vi "create.mcap_id.vi"(10 "id":i32) -> (3 "Timestamp Manifest":refnum<class "mcap.lvclass">)   [LabVIEW 2020, in "nominal types.lvlib" / "timestampManifest.lvlib"]
uses:
  timestampManifest.lvlib
  mcap/mcap.lvclass
  id/id.lvclass
  C:/code/labview-client/lv_src/nominal types/filterTypes/filterTypes.lvclass
  C:/code/labview-client/lv_src/Nominal Client/datasources/payload/payload.lvclass
  C:/code/labview-client/lv_src/nominal types/id/id.lvclass
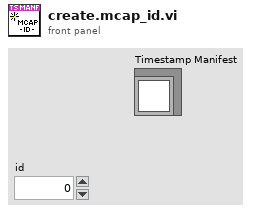
[diagram p1: front panel]
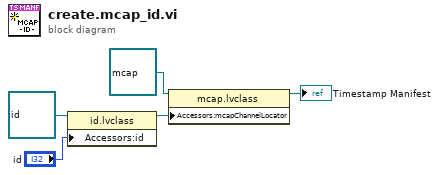
[diagram p0: block diagram]
diagram:
  n1 = property class="id.lvclass"(reference=refnum<class "id.lvclass"> refnum ("nominal types.lvlib:channelFilter.lvlib:id.lvclass"), "Accessors:id"="id") -> (reference out=w2:refnum<class "id.lvclass">)  [unwired: 1 in, 1 out]
  n2 = property class="mcap.lvclass"(reference=refnum<class "mcap.lvclass"> refnum ("nominal types.lvlib:timestampManifest.lvlib:mcap.lvclass"), "Accessors:mcapChannelLocator"=w2) -> (reference out=→"Timestamp Manifest":refnum<class "mcap.lvclass">)  [unwired: 1 in, 1 out]
